vi "create Haeuser.vi"() -> (3 "Häuser":cluster{i32[][]}[](array[cluster]))   [LabVIEW 2019]
uses:
  <vilib>/Analysis/baseanly.llb/Real A x B.vi
  <vilib>/Analysis/NI_AALBase.lvlib
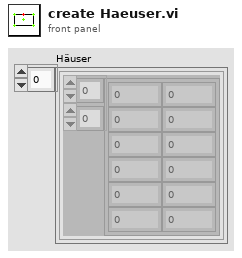
[diagram p1: front panel]
types:
  T1 = typedef "NI_Matrix.lvlib/RealMatrix.ctl" = dbl[][]
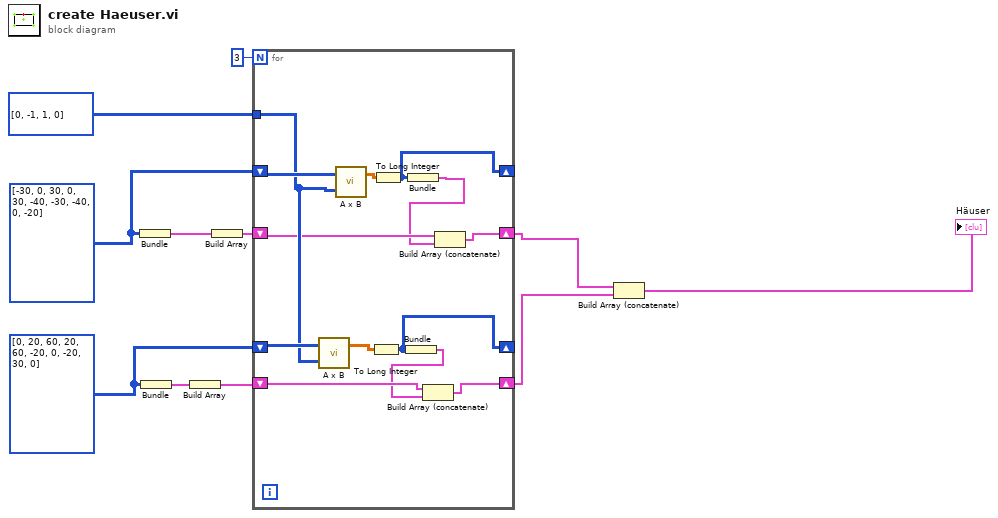
[diagram p0: block diagram]
diagram:
  w4 = i32[][] [[0, 20], [60, 20], [60, -20], [0, -20], [30, 0]]
  w5 = i32[][] [[-30, 0], [30, 0], [30, -40], [-30, -40], [0, -20]]
  n1 = Bundle(w5) -> (w2:cluster{i32[][]})  [unwired: 1 in]
  n2 = Bundle(w4) -> (w3:cluster{i32[][]})  [unwired: 1 in]
  n3 = Build Array(w3) -> (w8:cluster{i32[][]}[])
  n4 = Build Array(w2) -> (w7:cluster{i32[][]}[])
  n5 = for {
    N: 3 -> [_]
    shift-right: [w18] -> w10
    shift-left: w7 -> [w19]
    shift-right: [w13] -> w9
    shift-left: w8 -> [w15]
    shift-right: [w16] -> _
    shift-left: w5 -> [w24]
    shift-right: [w12] -> _
    shift-left: w4 -> [w23]
    tunnel: i32[][] [[0, -1], [1, 0]] -> [w22]
    n6 = call-poly <vilib>:"A x B.vi"("B"=w22, "A"=w23) -> ("A x B"=w20:T1)  [unwired: 1 out]
    n7 = call-poly <vilib>:"A x B.vi"("B"=w22, "A"=w24) -> ("A x B"=w21:T1)  [unwired: 1 out]
    n8 = To Long Integer(number=w20) -> (32bit integer=w12:i32[][])
    n9 = To Long Integer(number=w21) -> (32bit integer=w16:i32[][])
    n10 = Bundle(w12) -> (w14:cluster{i32[][]})  [unwired: 1 in]
    n11 = Bundle(w16) -> (w17:cluster{i32[][]})  [unwired: 1 in]
    n12 = Build Array (concatenate)(w15, w14) -> (w13:cluster{i32[][]}[])
    n13 = Build Array (concatenate)(w19, w17) -> (w18:cluster{i32[][]}[])
  }
  n14 = Build Array (concatenate)(w10, w9) -> (→"Häuser":cluster{i32[][]}[])
